vi "set channels.vi"(8 "error in (no error)":errorcluster, 10 "channels":refnum<class "TBM channel.lvclass">[](array[class]), 11 "module configuration in":refnum<class "tag select module configuration.lvclass">) -> (0 "error out":errorcluster, 3 "module configuration out":refnum<class "tag select module configuration.lvclass">)   [LabVIEW 2015, in "tag select module configuration.lvclass"]
uses:
  tag select module configuration.lvclass
  <vilib>/NI/Tag Bus Module Framework/channel/TBM channel.lvclass
  tag select module configuration.lvclass/tag select module configuration.ctl
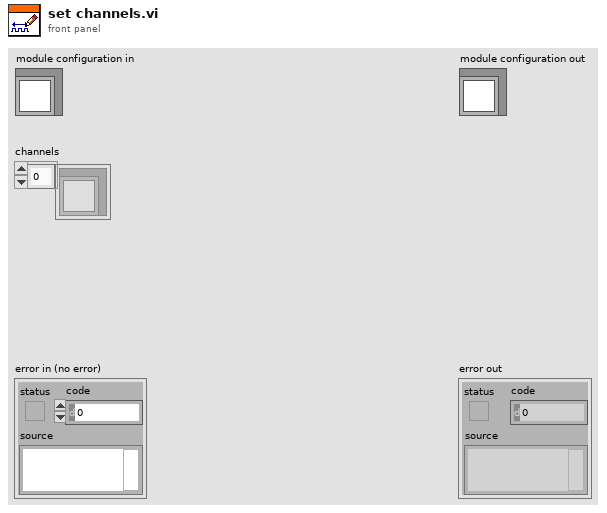
[diagram p1: front panel]
types:
  T1 = typedef "tag select module configuration.lvclass/tag select configuration.ctl" = cluster{"tag select name":string, "data type":T2, "output":refnum<class "TBM channel.lvclass">, "select":refnum<class "TBM channel.lvclass">, "input channels":refnum<class "TBM channel.lvclass">[]}
  T2 = typedef "tag bus.lvlib/tag descriptor.lvclass/Data Type.ctl" = enum16{"Double", "Single", "I64", "I32", "I16", "I8", "U64", "U32", "U16", "U8", "Boolean", "String", "Array of Double", "Array of Single", "Array of I64", "Array of I32", "Array of I16", "Array of I8", "Array of U64", "Array of U32", "Array of U16", "Array of U8", "Array of Boolean", "Array of String"}
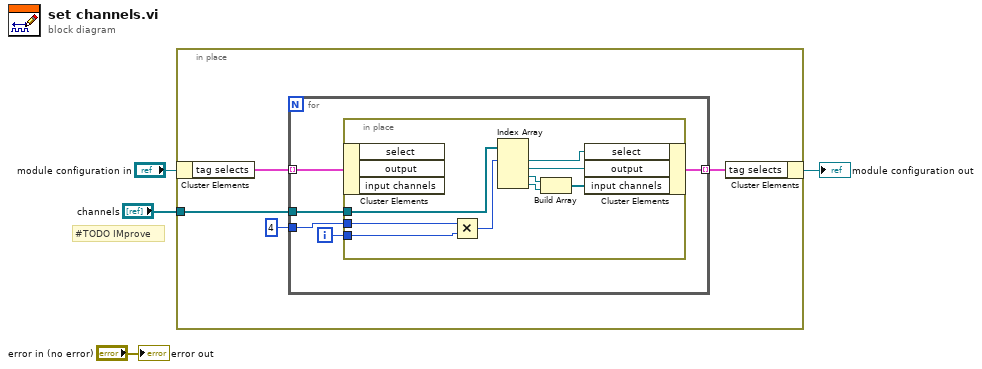
[diagram p0: block diagram]
diagram:
  # "#TODO IMprove"
  n1 = in-place {
    in-place-border: "channels" -> [w7]
    n2 = in-place-cluster #1("module configuration in") -> ("tag selects"=w8:T1[])
    n3 = for {
      tunnel: w8 -> [w10] mode=indexing
      tunnel: w7 -> [w13]
      tunnel: 4 -> [w11]
      tunnel: [w9] -> w5 mode=indexing
      i -> [w12]
      n4 = in-place {
        in-place-border: w13 -> [w19]
        in-place-border: w12 -> [w22]
        in-place-border: w11 -> [w21]
        n5 = in-place-cluster #2(w10) -> ()  [unwired: 3 out]
        n6 = Multiply(x=w21, y=w22) -> (x*y=w20:i32)
        n7 = Index Array(array=w19, index #1=w20) -> (element #1=w18:refnum<class "TBM channel.lvclass">, element #2=w17:refnum<class "TBM channel.lvclass">, element #3=w16:refnum<class "TBM channel.lvclass">, element #4=w15:refnum<class "TBM channel.lvclass">)  [unwired: 3 in]
        n8 = Build Array(w16, w15) -> (w14:refnum<class "TBM channel.lvclass">[])
        n9 = in-place-cluster #2("select"=w18, "output"=w17, "input channels"=w14) -> (w9:T1)
      }
    }
    n10 = in-place-cluster #1("tag selects"=w5) -> (→"module configuration out":refnum<class "tag select module configuration.lvclass">)
  }
  "error out" <- "error in (no error)"
